vi "Integration Reset.vi"(8 "error in (no error)":errorcluster, 10 "Card #":u8, 11 "Yokogawa WT500 in":refnum<class "Yokogawa WT500.lvclass">) -> (0 "error out":errorcluster, 3 "Yokogawa WT500 out":refnum<class "Yokogawa WT500.lvclass">)   [LabVIEW 2013, in "Generic Power Analyzer.lvlib" / "Yokogawa WT500.lvlib" / "Yokogawa WT500.lvclass"]
uses:
  Yokogawa WT500.lvclass
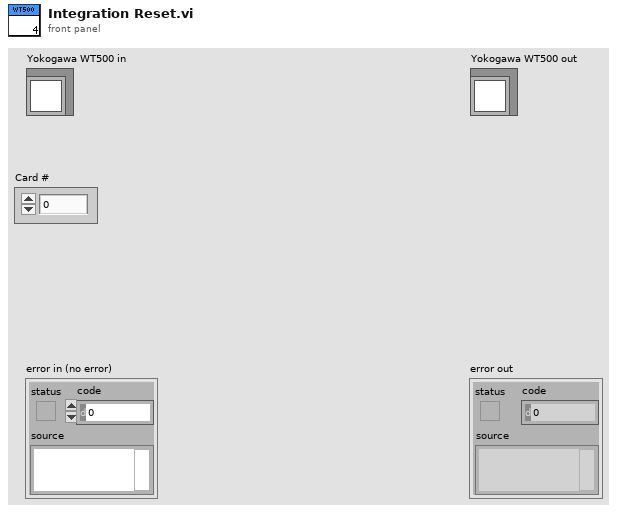
[diagram p1: front panel]
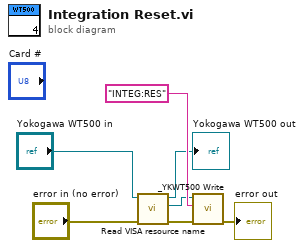
[diagram p0: block diagram]
diagram:
  n1 = call-dynamic "Read VISA resource name.vi"("error in (no error)"="error in (no error)", "Generic Instrument in"="Yokogawa WT500 in") -> ("error out"=w2:errorcluster, "VISA resource name"=w3:refnum<visa-resource-name>, "Generic Instrument out"=→"Yokogawa WT500 out":refnum<class "Yokogawa WT500.lvclass">)  [unwired: 7 in]
  n2 = call <instrlib>:"_YKWT500 Write.vi"("error in (no error)"=w2, "Write Data"="INTEG:RES", "VISA resource name"=w3) -> ("error out"=→"error out":errorcluster)  [unwired: 5 in, 3 out]
